vi "Launch Load Configuration.vi"(8 "error in":errorcluster, 11 "Master Controller in":refnum<class "EMS User Interface.lvclass">) -> (0 "error out":errorcluster, 3 "Master Controller out":refnum<class "EMS User Interface.lvclass">)   [LabVIEW 2018, in "EMS User Interface Actor.lvlib" / "EMS User Interface.lvclass"]
uses:
  EMS User Interface.lvclass
  C:/Program Files (x86)/National Instruments/LabVIEW 2018/vi.lib/ActorFramework/Actor/Actor.lvclass
  C:/Users/Administrator/Desktop/2018LabVIEW EMS/EMS Generic Actor/EMS Generic/EMS Generic.lvclass
  Dialog Actors/File Dialog Actor/File Dialog/File Dialog.lvclass
  EMS User Interface Messages/Configuration Load Msg/Configuration Load Msg.lvclass
  C:/Users/Administrator/Desktop/2018LabVIEW EMS/Dialog Actors/File Dialog Actor/File Dialog Messages/Return File Path Msg/Return File Path Msg.lvclass
  EMS Generic Actor/EMS Generic/EMS Generic.lvclass/EMS Generic.ctl
  Dialog Actors/File Dialog Actor/File Dialog/File Dialog.lvclass/File Dialog.ctl
  <vilib>/ActorFramework/Actor/Actor.lvclass
  EMS Generic Actor/EMS Generic/EMS Generic.lvclass
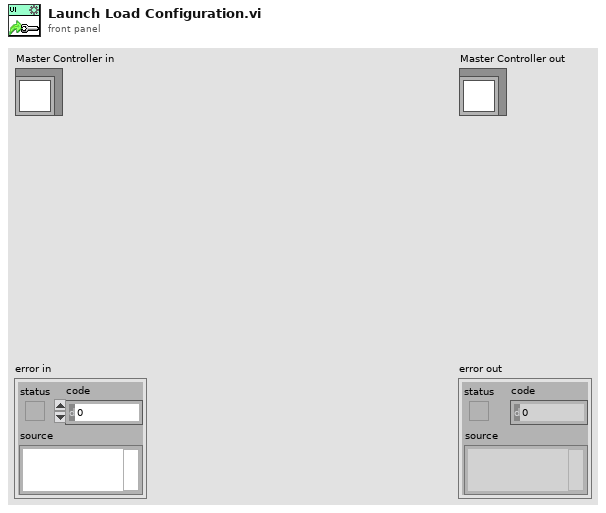
[diagram p1: front panel]
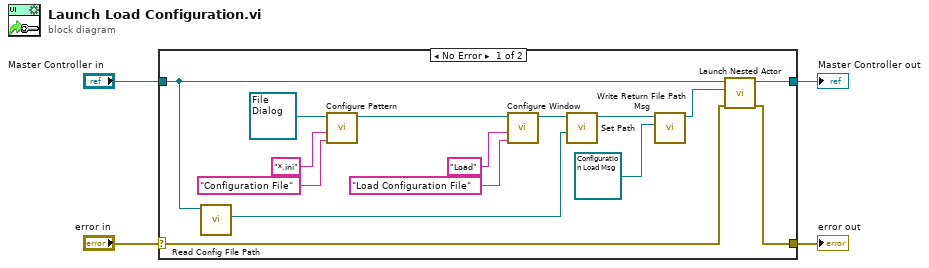
[diagram p0: block diagram]
diagram:
  n1 = case shown="No Error" "error in" {
    selector: "error in" -> [w9 w21]
    tunnel: [w8 w21] -> w3
    tunnel: [w11 w20] -> w1
    tunnel: "Master Controller in" -> [w6 w20]
    frame No Error {
      n2 = call "Read Config File Path.vi"("EMS Generic in"=w6) -> ("Config File Path"=w5:path)  [unwired: 8 in, 2 out]
      n3 = call "Configure Pattern.vi"("Pattern Label"="Configuration File", "Pattern"="*.ini", "File Dialog in"=refnum<class "File Dialog.lvclass"> refnum ("File Dialog Actor.lvlib:File Dialog.lvclass")) -> ("File Dialog out"=w19:refnum<class "File Dialog.lvclass">)  [unwired: 8 in]
      n4 = call "Configure Window.vi"("Prompt"="Load Configuration File" ("Pattern Label"), "Button Label"="Load" ("Pattern"), "File Dialog in"=w19) -> ("File Dialog out"=w17:refnum<class "File Dialog.lvclass">)  [unwired: 8 in]
      n5 = call "Set Path.vi"("Path"=w5, "File Dialog in"=w17) -> ("File Dialog out"=w16:refnum<class "File Dialog.lvclass">)  [unwired: 9 in]
      n6 = call "Write Return File Path Msg.vi"("Return File Path Msg"=refnum<class "Configuration Load Msg.lvclass"> refnum ("Master Controller Core.lvlib:Configuration Load Msg.lvclass"), "File Dialog in"=w16) -> ("File Dialog out"=w10:refnum<class "File Dialog.lvclass">)  [unwired: 9 in]
      n7 = call <vilib>:"Launch Nested Actor.vi"("error in (no error)"=w9, "Nested Actor"=w10, "Caller Actor in"=w6) -> ("error out"=w8:errorcluster, "Caller Actor out"=w11:refnum<class "EMS User Interface.lvclass">)  [unwired: 6 in, 1 out]
    }
    frame Error {
    }
  }
  "error out" <- w3
  "Master Controller out" <- w1
